vi "Keithley SubVI.vi"() -> ()   [LabVIEW 2013]
uses:
  <vilib>/Instr/_visa.llb/VISA Configure Serial Port (Instr).vi
panel:
  out "Resistivity":dbl
  in  "Correction Factor":dbl=1.0
  in  "Thickness (in nm)":dbl=1.0
  out "Resistivity Graph":cluster{dbl[], dbl[]}(graph)
  out "Current Graph":cluster{dbl[], dbl[]}(graph)
  out "Voltage Graph":cluster{dbl[], dbl[]}(graph)
  in  "Unit   2":string(combo)="1"
  out "Current":string
  out "Voltage":string
  out "read buffer":string
  in  "Voltage Protection":dbl
  in  "Unit":string(combo)="2"
  in  "Current":dbl
  in  "flow control (0:none)":u16(ring) items=["None", "XON/XOFF", "RTS/CTS", "XON/XOFF & RTS/CTS", "DTR/DSR", "XON/XOFF & DTR/DSR"]
  in  "stop bits (10: 1 bit)":u16(ring)=10 items=["1.0"=10, "1.5"=15, "2.0"=20]
  in  "parity (0:none)":enum16{"None", "Odd", "Even", "Mark", "Space"}(ring)
  in  "data bits (8)":u16=8 min=5 max=8 step=1
  in  "baud rate (9600)":u32=9600
  in  "VISA resource name 2":refnum<visa-resource-name>="COM1"
  # "nm"
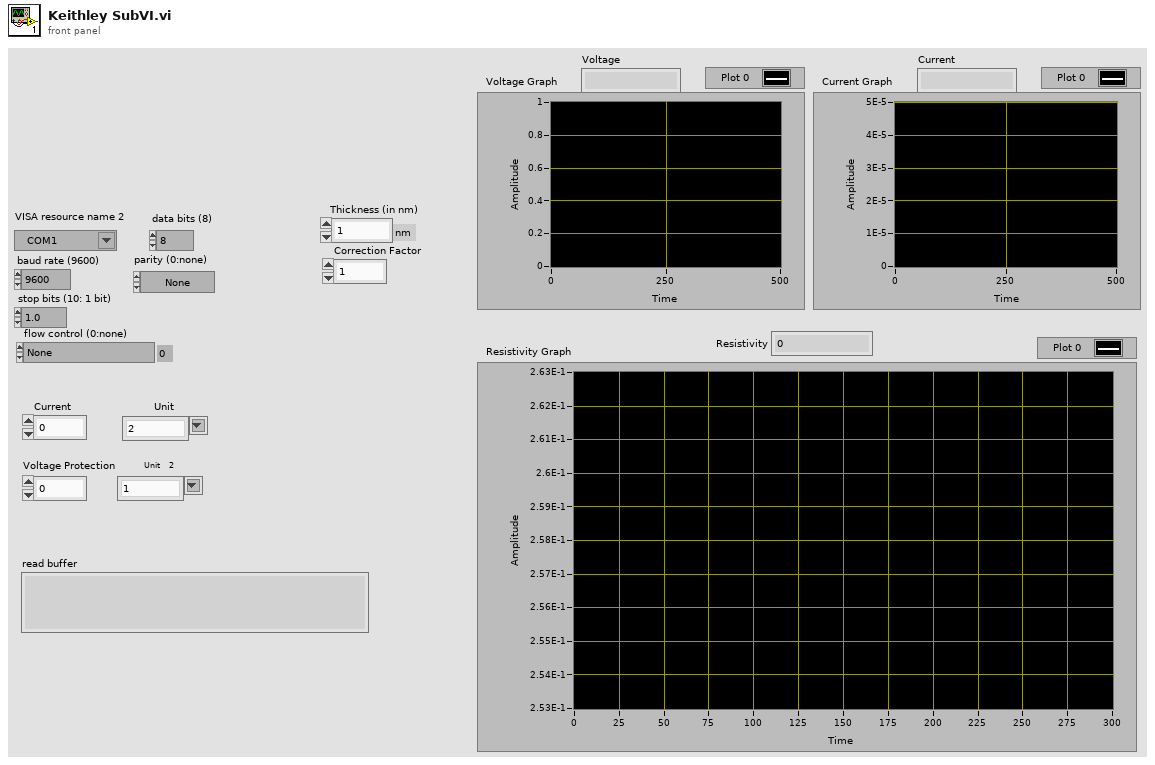
[diagram p1: front panel]
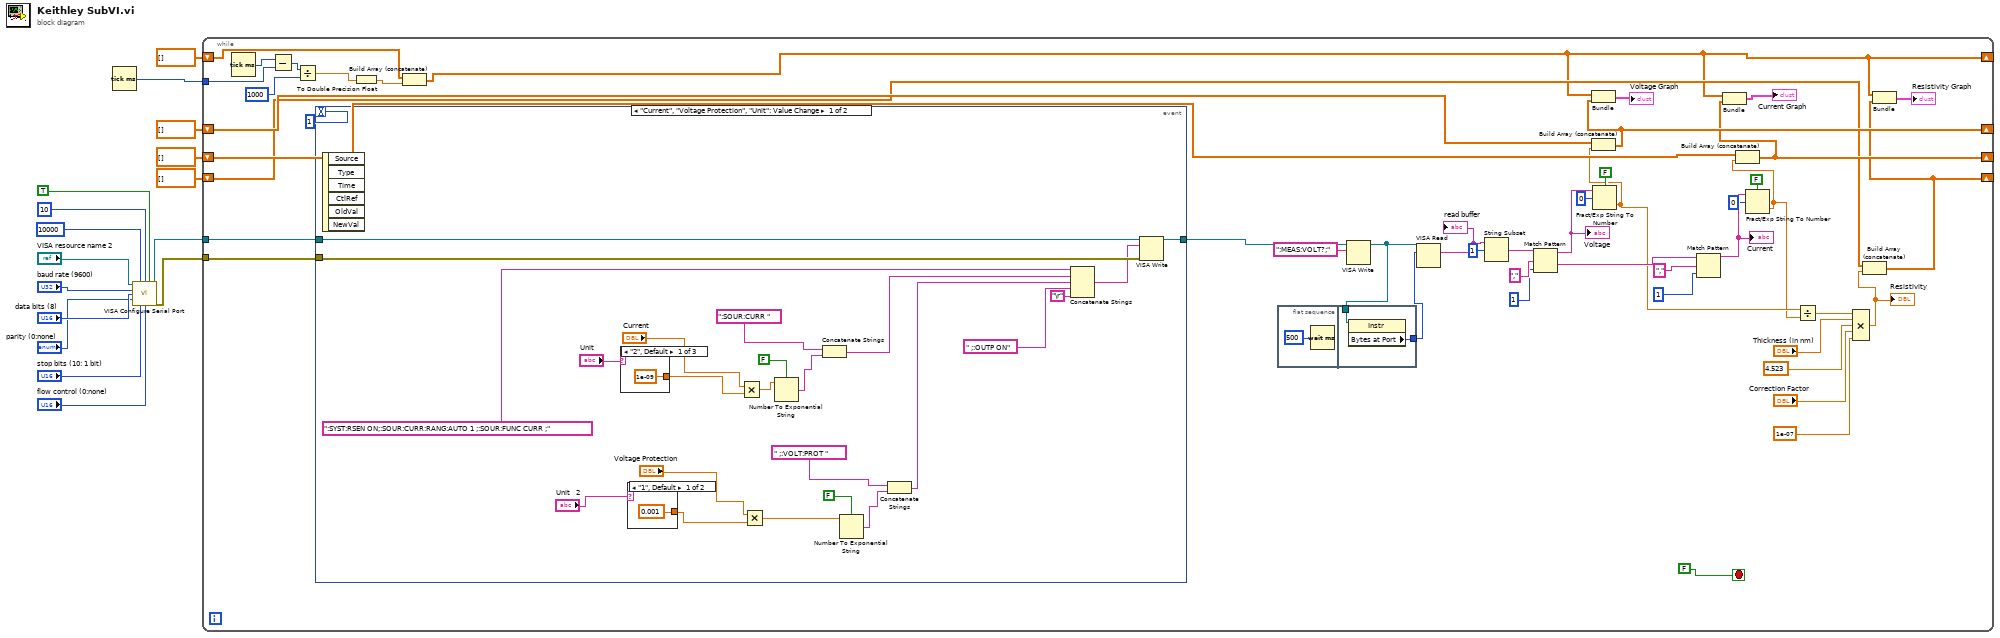
[diagram p0: block diagram]
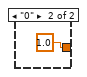
[diagram p2: hidden frame]
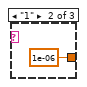
[diagram p3: hidden frame]
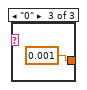
[diagram p4: hidden frame]
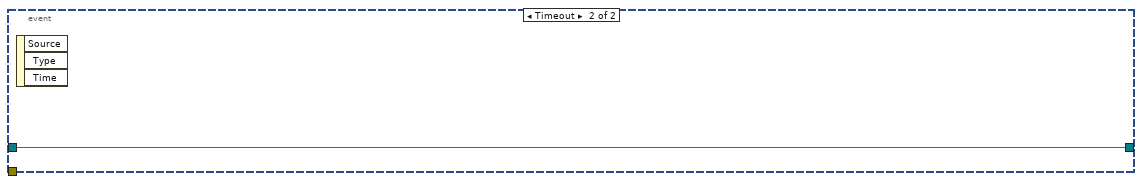
[diagram p5: hidden frame]
diagram:
  n1 = Tick Count (ms)() -> (millisecond timer value=w4:u32)
  n2 = call-poly "VISA Configure Serial Port"("VISA resource name"="VISA resource name 2", "timeout (10sec)"=u32 10000, "termination char\n(0xA = '\\n' = LF)"=u8 10 ("termination char\n(0xA = '\\n' = LF)"), "Enable Termination\nChar (T)"=TRUE ("Enable Termination\nChar (T)"), "baud rate (9600)"="baud rate (9600)", "data bits (8)"="data bits (8)", "parity (0:none)"="parity (0:none)", "stop bits (10: 1 bit)"="stop bits (10: 1 bit)", "flow control (0:none)"="flow control (0:none)") -> ("VISA resource name out"=w7:refnum<visa-resource-name>, "error out"=w6:errorcluster)  [unwired: 5 in]
  n3 = while {
    tunnel: w7 -> [w63]
    tunnel: w6 -> [w62]
    shift-right: [w19] -> _
    shift-left: dbl[] [] -> [w46]
    shift-right: [w43] -> _
    shift-left: dbl[] [] -> [w44]
    shift-right: [w39] -> _
    shift-left: dbl[] [] -> [w40]
    tunnel: w4 -> [w33]
    shift-right: [w18] -> _
    shift-left: dbl[] [] -> [w22]
    stop <- FALSE stop-if-true
    n4 = Tick Count (ms)() -> (millisecond timer value=w34:u32)
    n5 = Subtract(x=w34, y=w33) -> (x-y=w35:u32)
    n6 = Divide(x=w35, y=1000) -> (x/y=w37:dbl)
    n7 = event shown="[0] \"Current\", \"Voltage Protection\", \"Unit\": Value Change" {
      selector: _ -> [_ _]
      dyn-events: _ -> [_ _]
      timeout: 1 -> [_ _]
      tunnel: w63 -> [w86 w92]
      tunnel: w62 -> [w85 _]
      tunnel: [w84 w92] -> w61
      event "Current", "Voltage Protection", "Unit": Value Change {
        n8 = event-data() -> ()  [unwired: 1 in, 6 out]
        n9 = case shown="\"2\", Default" "Unit" {
          tunnel: [1e-09 ("y") 1e-06 ("y") 0.001 ("y")] -> w71
          frame "2", Default {
          }
          frame "1" {
          }
          frame "0" {
          }
        }
        n10 = case shown="\"1\", Default" "Unit   2" {
          tunnel: [0.001 ("y") 1.0 ("y")] -> w67
          frame "1", Default {
          }
          frame "0" {
          }
        }
        n11 = Multiply(x="Current", y=w71) -> (x*y=w74:dbl)
        n12 = Multiply(x="Voltage Protection", y=w67) -> (x*y=w65:dbl)
        n13 = Number To Exponential String(number=w74, 1:FALSE ("use system decimal point (T)")) -> (E-format string=w76:string)  [unwired: 2 in]
        n14 = Concatenate Strings(":SOUR:CURR " ("string"), w76) -> (w82:string)
        n15 = Number To Exponential String(number=w65, 1:FALSE ("use system decimal point (T)")) -> (E-format string=w69:string)  [unwired: 2 in]
        n16 = Concatenate Strings(" ;:VOLT:PROT " ("string"), w69) -> (w81:string)
        n17 = Concatenate Strings(":SYST:RSEN ON;:SOUR:CURR:RANG:AUTO 1 ;:SOUR:FUNC CURR ;" ("write buffer"), w82, w81, " ;:OUTP ON" ("string"), "\r") -> (w80:string)
        n18 = VISA Write(VISA resource name=w86, write buffer=w80, error in (no error)=w85) -> (VISA resource name out=w84:refnum<visa-resource-name>)  [unwired: 2 out]
      }
      event Timeout {
        n19 = event-data() -> ()  [unwired: 1 in, 3 out]
      }
    }
    n20 = To Double Precision Float(number=w37) -> (double precision float=w36:dbl)
    n21 = Build Array (concatenate)(w46, w36) -> (w19:dbl[])
    n22 = flat-sequence {
      tunnel: [w95] -> w59
      tunnel: w58 -> [w94]
      frame #0 {
        n23 = Wait (ms)(milliseconds to wait=u32 500) -> ()  [unwired: 1 out]
      }
      frame #1 {
        n24 = property class="Instr"(reference=w94) -> ("Bytes at Port"=w95:u32)  [unwired: 1 in, 2 out]
      }
    }
    n25 = VISA Write(VISA resource name=w61, write buffer=":MEAS:VOLT?;") -> (VISA resource name out=w58:refnum<visa-resource-name>)  [unwired: 1 in, 2 out]
    n26 = VISA Read(VISA resource name=w58, byte count=w59) -> (read buffer=w52:string)  [unwired: 1 in, 3 out]
    "read buffer" <- w52
    n27 = String Subset(string=w52, offset (0)=1) -> (substring=w51:string)  [unwired: 1 in]
    n28 = Match Pattern(string=w51, regular expression=",", offset (0)=1) -> (before substring=w45:string, after substring=w53:string)  [unwired: 2 out]
    "Voltage" <- w45
    n29 = Fract/Exp String To Number(use system decimal point (T)=FALSE, string=w45, offset=0) -> (number=w28:dbl)  [unwired: 1 in, 1 out]
    n30 = Build Array (concatenate)(w44, w28) -> (w43:dbl[])
    n31 = Bundle(w19, w43) -> (→"Voltage Graph":cluster{dbl[], dbl[]})  [unwired: 1 in]
    n32 = Match Pattern(string=w53, regular expression=",", offset (0)=1) -> (before substring=w41:string)  [unwired: 3 out]
    "Current" <- w41
    n33 = Fract/Exp String To Number(use system decimal point (T)=FALSE, string=w41, offset=0) -> (number=w27:dbl)  [unwired: 1 in, 1 out]
    n34 = Build Array (concatenate)(w40, w27) -> (w39:dbl[])
    n35 = Bundle(w19, w39) -> (→"Current Graph":cluster{dbl[], dbl[]})  [unwired: 1 in]
    n36 = Divide(x=w28, y=w27) -> (x/y=w26:dbl)
    n37 = Compound Arithmetic op=MULTIPLY(w26, "Thickness (in nm)", 4.523 ("value"), "Correction Factor", 1e-07 ("value")) -> (w21:dbl)
    "Resistivity" <- w21
    n38 = Build Array (concatenate)(w22, w21) -> (w18:dbl[])
    n39 = Bundle(w19, w18) -> (→"Resistivity Graph":cluster{dbl[], dbl[]})  [unwired: 1 in]
  }
